vi "Discover and Search Temp.vi"() -> ()   [LabVIEW 2014]
panel:
  in  "Error In":errorcluster
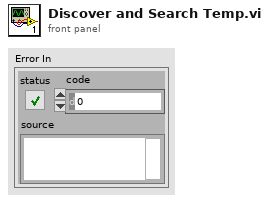
[diagram p1: front panel]
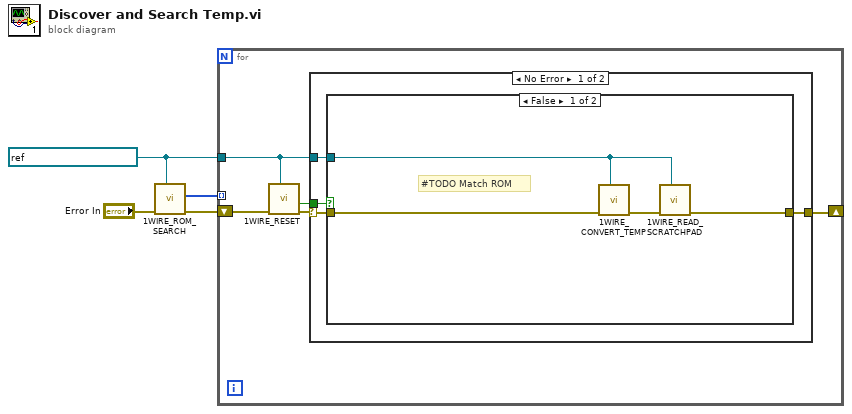
[diagram p0: block diagram]
diagram:
  w1 = refnum<k21> "ConnectorA/DIO15" ("1-Wire DIO Pin")
  n1 = call "1WIRE_ROM_SEARCH.vi"("1-Wire DIO Pin"=w1, "Error In"="Error In") -> ("Error Out"=w3:errorcluster, "ROM Array"=w2:u64[])  [unwired: 8 in]
  n2 = for {
    shift-right: [w5] -> _
    shift-left: w3 -> [w9]
    tunnel: w2 -> [_] mode=indexing
    tunnel: w1 -> [w6]
    n3 = call "1WIRE_RESET.vi"("1-Wire DIO Pin"=w6, "error in"=w9) -> ("error out"=w7:errorcluster, "0 = Device Present / 1=no"=w8:bool)  [unwired: 8 in]
    n4 = case shown="No Error" w7 {
      selector: w7 -> [w11 _]
      tunnel: w8 -> [w13 _]
      tunnel: w6 -> [w12 _]
      tunnel: [w10 _] -> w5
      frame No Error {
        n5 = case shown="False" w13 {
          tunnel: w12 -> [w14 _]
          tunnel: w11 -> [w17 _]
          tunnel: [w15 _] -> w10
          frame False {
            # "#TODO Match ROM"
            n6 = call "1WIRE_CONVERT_TEMP.vi"("1-Wire DIO Pin"=w14, "error in (no error)"=w17) -> ("error out"=w16:errorcluster)  [unwired: 8 in, 1 out]
            n7 = call "1WIRE_READ_SCRATCHPAD.vi"("1-Wire DIO Pin"=w14, "error in (no error)"=w16) -> ("error out"=w15:errorcluster)  [unwired: 7 in, 1 out]
          }
          frame True {
          }
        }
      }
      frame Error {
      }
    }
  }
